vi "Engine In - Sensor - EGR Valve Position.vi"(10 "Loop Freq (Hz)":sgl, 11 "EGR Valve Position [V]":sgl) -> (3 "EGR Valve Position [%]":sgl)   [LabVIEW 2015, in "ECS-RT.lvlib"]
uses:
  ECS-RT.lvlib
  <vilib>/ptbypt/NI_PtbyPt.lvlib
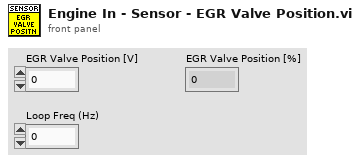
[diagram p1: front panel]
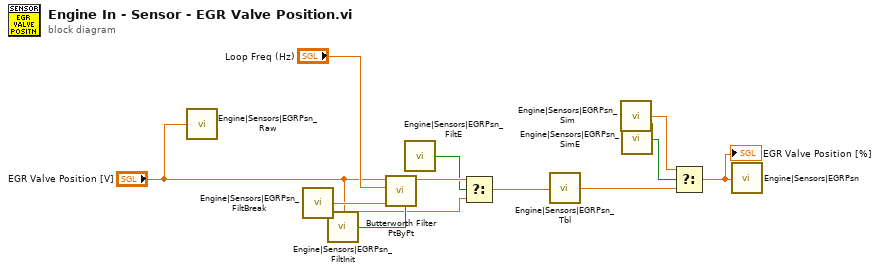
[diagram p0: block diagram]
diagram:
  n1 = call "Engine|Sensors|EGRPsn_Raw"("Value"="EGR Valve Position [V]") -> ()
  n2 = call "Engine|Sensors|EGRPsn_FiltBreak"() -> ("Value"=w7:sgl)
  n3 = call "Engine|Sensors|EGRPsn_FiltInit"() -> ("Value"=w10:bool)
  n4 = call <vilib>:"Butterworth Filter PtByPt.vi"("initialize"=w10, "low cutoff freq: fl"=w7, "sampling freq: fs"="Loop Freq (Hz)", "x"="EGR Valve Position [V]") -> ("Filtered x"=w9:dbl)  [unwired: 5 in, 1 out]
  n5 = call "Engine|Sensors|EGRPsn_FiltE"() -> ("Value"=w6:bool)
  n6 = Select(t=w9, s=w6, f="EGR Valve Position [V]") -> (s? t:f=w8:dbl)
  n7 = call "Engine|Sensors|EGRPsn_Tbl"("X Index"=w8) -> ("Y"=w5:sgl)
  n8 = call "Engine|Sensors|EGRPsn_Sim"() -> ("Value"=w11:sgl)
  n9 = call "Engine|Sensors|EGRPsn_SimE"() -> ("Value"=w4:bool)
  n10 = Select(t=w11, s=w4, f=w5) -> (s? t:f=w2:sgl)
  "EGR Valve Position [%]" <- w2
  n11 = call "Engine|Sensors|EGRPsn"("Value"=w2) -> ()
